vi "printLog.vi"(8 "error in (no error)":errorcluster, 11 "Log in":refnum<class "Log.lvclass">) -> (0 "error out":errorcluster, 2 "String":string, 3 "Log out":refnum<class "Log.lvclass">)   [LabVIEW 2011, in "Tools.lvlib" / "xml.lvlib" / "Log.lvclass"]
uses:
  Log.lvclass
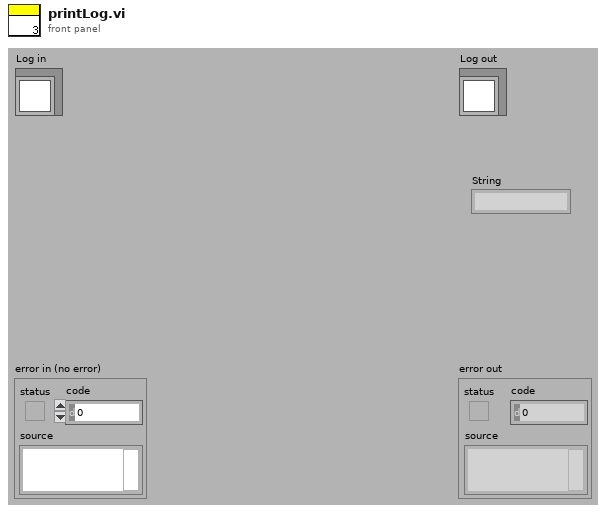
[diagram p1: front panel]
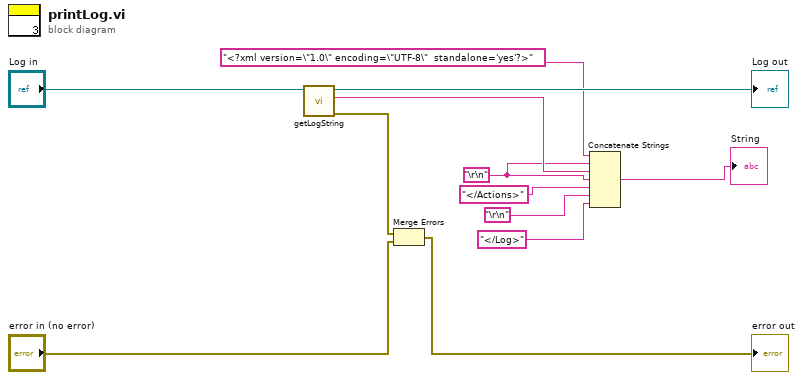
[diagram p0: block diagram]
diagram:
  w1 = "\r\n"
  n1 = call-dynamic "getLogString.vi"("Log.lvclass in"="Log in") -> ("error out"=w10:errorcluster, "logString"=w7:string, "Log.lvclass out"=→"Log out":refnum<class "Log.lvclass">)  [unwired: 8 in]
  n2 = Merge Errors(w10, "error in (no error)") -> (→"error out":errorcluster)
  n3 = Concatenate Strings("<?xml version=\"1.0\" encoding=\"UTF-8\"  standalone='yes'?>", w1, w7, w1, "</Actions>", "\r\n", "</Log>") -> (→"String":string)
